vi "FetchTemp34980.vi"(4 "error in (no error)":errorcluster, 7 "Circuit ID":i32=1019 format="%_4g") -> (0 "Error out":errorcluster, 1 "Temp C":dbl, 2 "Temp F":dbl, 3 "Voltage":dbl format="%#_10e")   [LabVIEW 2009]
doc: "Reads a value from the 34980 and then convert volts to temperature.\nAssumes that you have scanned the 34980 to store the values."
panel:
  # "This assumes you have already scanned the 34980"
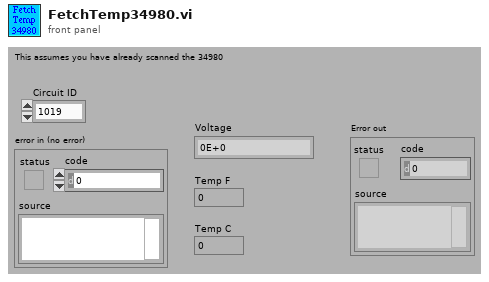
[diagram p1: front panel]
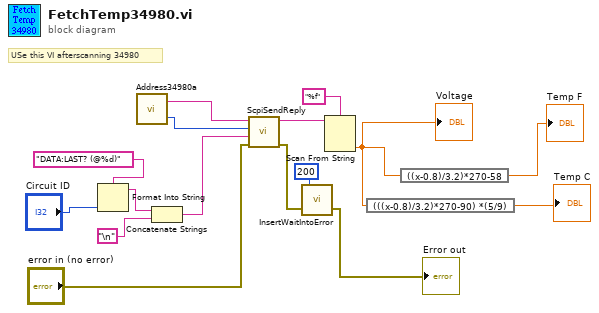
[diagram p0: block diagram]
diagram:
  # "USe this VI afterscanning 34980"
  n1 = Format Into String(format string="DATA:LAST? (@%d)", "Circuit ID") -> (resulting string=w9:string)  [unwired: 2 in, 1 out]
  n2 = call "Address34980a.vi"() -> ("Port"=w13:i32, "IP address"=w12:string)  [unwired: 2 in]
  n3 = Concatenate Strings(w9, "\n") -> (w7:string)
  n4 = call "ScpiSendReply.vi"("error in (no error)"="error in (no error)", "Command"=w7, "TCP port"=w13, "IP Address"=w12) -> ("Error out"=w6:errorcluster, "Reply"=w15:string)  [unwired: 5 in]
  n5 = call "InsertWaitIntoError.vi"("error in (no error)"=w6, "Wait (msecs)"=200) -> ("error out"=→"Error out":errorcluster)  [unwired: 1 in]
  n6 = Scan From String(format string="%f", input string=w15) -> (output 1=w1:dbl)  [unwired: 3 in, 3 out]
  "Voltage" <- w1
  n7 = expression code="(((x-0.8)/3.2)*270-90) *(5/9)"(w1) -> (→"Temp C":dbl)
  n8 = expression code="((x-0.8)/3.2)*270-58"(w1) -> (→"Temp F":dbl)
